vi "holoComp2.vi"(7 "Beam Parameters, dependant on SLM and LASER  B":T2={"amplitude matrix"=[], "number of columns in amplitude matrix"=1400, "number of rows in amplitude matrix"=1050, "represented width (in m)"=0.01498, "represented height (in m)"=0.01092, "wavelength (in m)"=6.33e-07}, 8 "No.of Quadrants":i32=6 min=0 max=90, 9 "Pie Cut Weighting":T1 {"1" min=0.0 max=360.0 step=180.0; "2" min=0.0 max=360.0 step=180.0; "3" min=0.0 max=360.0 step=180.0; "4" min=0.0 max=360.0 step=180.0; "5" min=0.0 max=360.0 step=180.0; "6" min=0.0 max=360.0 step=180.0}, 10 "Pie cut separation (degrees)":i32=5 max=90, 11 "hologramIn":sgl[][](array[numeric])) -> (2 "holoAGrayscale":dbl[][](array[numeric]), 3 "Pie Cut Out":dbl[][](graph))   [LabVIEW 2020]
uses:
  <vilib>/express/express arith-compare/Formula/XNode/ExpressFormulaBlockNode.xnode
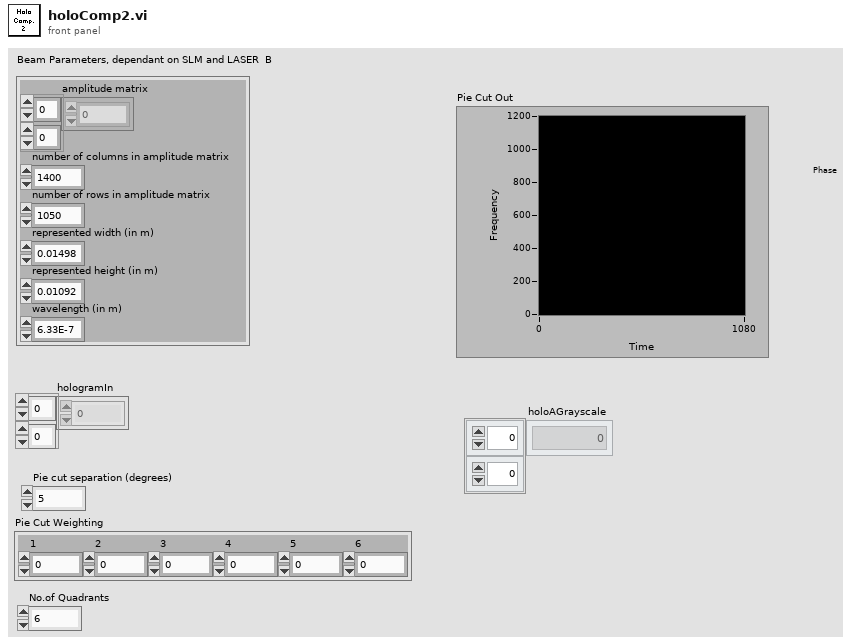
[diagram p1: front panel]
types:
  T1 = cluster{"1":dbl, "2":dbl, "3":dbl, "4":dbl, "5":dbl, "6":dbl}
  T2 = cluster{"amplitude matrix":csg[][], "number of columns in amplitude matrix":i32, "number of rows in amplitude matrix":i32, "represented width (in m)":dbl, "represented height (in m)":dbl, "wavelength (in m)":dbl}
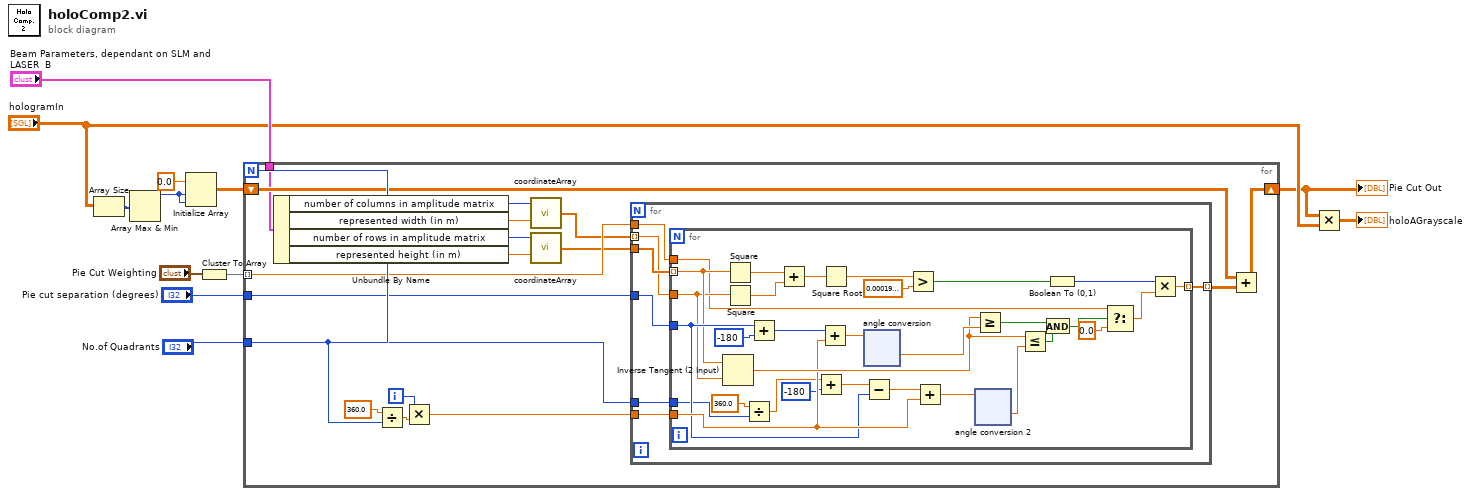
[diagram p0: block diagram]
diagram:
  n1 = Array Size(array="hologramIn") -> (size(s)=w10:i32[])
  n2 = Array Max & Min(array=w10) -> (max value=w9:i32)  [unwired: 3 out]
  n3 = Initialize Array(0.0 ("element"), w9, w9) -> (w12:dbl[][])
  n4 = Cluster To Array(cluster="Pie Cut Weighting") -> (array=w2:dbl[])
  n5 = for {
    N: "No.of Quadrants" -> [_]
    shift-right: [w24] -> w1
    shift-left: w12 -> [w25]
    tunnel: "Pie cut separation (degrees)" -> [w16]
    tunnel: "No.of Quadrants" -> [w14]
    tunnel: w2 -> [w19] mode=indexing
    tunnel: "Beam Parameters, dependant on SLM and LASER  B" -> [w20]
    i -> [w21]
    n6 = Unbundle By Name(w20) -> ("number of columns in amplitude matrix"=w29:i32, "represented width (in m)"=w28:dbl, "number of rows in amplitude matrix"=w27:i32, "represented height (in m)"=w26:dbl)
    n7 = Divide(x=360.0, y=w14) -> (x/y=w22:dbl)
    n8 = Multiply(x=w21, y=w22) -> (x*y=w15:dbl)
    n9 = call "coordinateArray.vi"("width of represented x (or y) range (in m; default 1E-3=1mm)"=w28, "array size (default 64)"=w29) -> ("x array"=w18:sgl[])
    n10 = call "coordinateArray.vi"("width of represented x (or y) range (in m; default 1E-3=1mm)"=w26, "array size (default 64)"=w27) -> ("x array"=w17:sgl[])
    n11 = for {
      tunnel: w17 -> [w36]
      tunnel: w18 -> [w35] mode=indexing
      tunnel: [w34] -> w13 mode=indexing
      tunnel: w15 -> [w33]
      tunnel: w16 -> [w32]
      tunnel: w14 -> [w31]
      tunnel: w19 -> [w30]
      n12 = for {
        tunnel: w36 -> [w48] mode=indexing
        tunnel: w35 -> [w46]
        tunnel: [w38] -> w34 mode=indexing
        tunnel: w33 -> [w59]
        tunnel: w32 -> [w55]
        tunnel: w31 -> [w53]
        tunnel: w30 -> [w37]
        n13 = Inverse Tangent (2 Input)(1:w46, 2:w48) -> (0:w61:sgl)
        n14 = Square(x=w48) -> (x^2=w47:sgl)
        n15 = Square(x=w46) -> (x^2=w45:sgl)
        n16 = Divide(x=360.0, y=w53) -> (x/y=w51:dbl)
        n17 = Add(x=w55, y=-180) -> (x+y=w57:i32)
        n18 = Add(x=w47, y=w45) -> (x+y=w44:sgl)
        n19 = Add(x=w51, y=-180) -> (x+y=w49:dbl)
        n20 = Add(x=w57, y=w59) -> (x+y=w60:dbl)
        n21 = Square Root(x=w44) -> (sqrt(x)=w43:sgl)
        n22 = xnode "angle conversion"("X1"=w60) -> ("Result"=w63:dbl)  [unwired: 1 in, 1 out]
        n23 = Subtract(x=w49, y=w55) -> (x-y=w56:dbl)
        n24 = Greater?(x=w43, y=sgl 0.0002) -> (0:w41:bool)
        n25 = Add(x=w56, y=w59) -> (x+y=w58:dbl)
        n26 = Greater Or Equal?(x=w61, y=w63) -> (x >= y?=w67:bool)
        n27 = xnode "angle conversion 2"("X1"=w58) -> ("Result"=w62:dbl)  [unwired: 1 in, 1 out]
        n28 = Less Or Equal?(x=w61, y=w62) -> (x <= y?=w66:bool)
        n29 = And(x=w67, y=w66) -> (x .and. y?=w65:bool)
        n30 = Boolean To (0,1)(Boolean=w41) -> (0, 1=w39:i16)
        n31 = Select(t=w37, s=w65, f=0.0) -> (s? t:f=w40:dbl)
        n32 = Multiply(x=w39, y=w40) -> (x*y=w38:dbl)
      }
    }
    n33 = Add(x=w25, y=w13) -> (x+y=w24:dbl[][])
  }
  "Pie Cut Out" <- w1
  n34 = Multiply(x=w1, y="hologramIn") -> (x*y=→"holoAGrayscale":dbl[][])
